vi "Check for Changes.vi"(11 "History":refnum<class "History.lvclass">) -> (2 "Have Changes":bool)   [LabVIEW 2020, in "lv_icon.lvlib" / "History.lvlib" / "History.lvclass"]
doc: "Checks if there were changes based on the history."
uses:
  History.lvclass
  History.lvclass/History.ctl
  History.lvlib
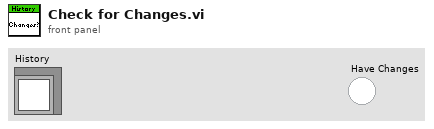
[diagram p1: front panel]
types:
  T1 = typedef "lv_icon.lvlib/History.lvlib/State.ctl" = cluster{"Template":string, "Layers":string, "Body Text":string, "Icon Text Layer":string, "Template Layer":string, "Templates Search":string, "Glyphs Search":string}
  T2 = cluster{"Template":bool, "Layers":bool, "Body Text":bool, "Icon Text Layer":bool, "Template Layer":bool, "Templates Search":bool, "Glyphs Search":bool}
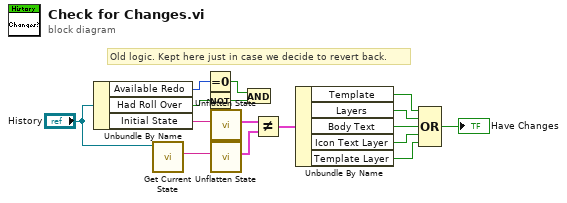
[diagram p0: block diagram]
diagram:
  # "Old logic. Kept here just in case we decide to revert back."
  n1 = Unbundle By Name("History") -> ("Available Redo"=w4:i32, "Had Roll Over"=w2:bool, "Initial State"=w14:string)
  n2 = call "Get Current State.vi"("History"="History") -> ("Current State"=w15:string)  [unwired: 8 in, 2 out]
  n3 = Equal To 0?(x=w4) -> (x = 0?=w3:bool)
  n4 = Not(x=w2) -> (.not. x?=w1:bool)
  n5 = call "Unflatten State.vi"("Flattened State"=w14) -> ("State"=w13:T1)  [unwired: 9 in, 1 out]
  n6 = call "Unflatten State.vi"("Flattened State"=w15) -> ("State"=w12:T1)  [unwired: 9 in, 1 out]
  n7 = And(x=w3, y=w1) -> ()  [unwired: 1 out]
  n8 = Not Equal?(x=w13, y=w12) -> (x != y?=w11:T2)
  n9 = Unbundle By Name(w11) -> ("Template"=w10:bool, "Layers"=w9:bool, "Body Text"=w8:bool, "Icon Text Layer"=w7:bool, "Template Layer"=w6:bool)
  n10 = Compound Arithmetic op=OR(w10, w9, w8, w7, w6) -> (→"Have Changes":bool)
